vi "JKISM++ Register Status Change.vi"(0 "JKISM Name":string, 5 "Source JKISM Name (* as Default)":string="*", 7 "Status":string, 9 "Response Message (if \"\", same as Source Message)":string, 11 "Error in":errorcluster caption="Error in (no error)", 12 "Priority(T:As Status,F:As Interrupt)":T1) -> (4 "JKISM Name(dup)":string, 15 "Error out":errorcluster)   [LabVIEW 2014, in "JKI State Machine++.lvlib"]
doc: "Register for notification of other JKISM++ Module's status change. If \"Response Message\" is not connected or \"\" is the input, the same state name will be used for acting message.\n\n<b>Inputs:</b>\n - <b>JKISM Name</b>: JKISM Module name.\n - <b>Source JKISM Name (* as Default)</b>: JKISM who generates the status. You can use '*' for all modules generated the same <b>Status</b>\n - <b>Status</b>: The status string\n - <b>Response Message (if \"\", same as Source Message)</b>: After registered, If status change, this message will be received.\n - <b>Priority(T:As Status,F:As Interrupt)</b>: The Response Message will be inserted to the front of state queue if it's False, otherwise it wil be append to the tail.\n - <b>Error in</b>: Error cluster\n\n<b>Outputs:</b>\n - <b>JKISM Name(dup)</b>: Return <b>JKISM Name</b>\n - <b>Error out</b>: Error cluster"
uses:
  JKI State Machine++.lvlib
  JKISM++ Broadcast Message Type.ctl
  _Support/FGV-BroadcastRegistry/Operation-BroadcastRegistry.ctl
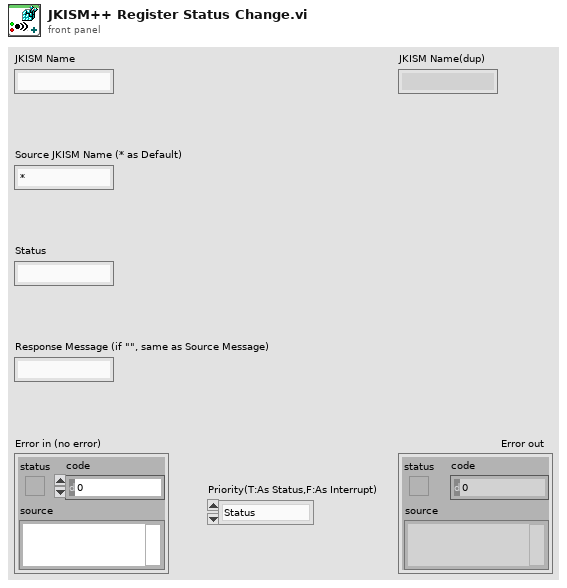
[diagram p1: front panel]
types:
  T1 = typedef "JKI State Machine++.lvlib/JKISM++ Broadcast Message Type.ctl" = enum16{"Status", "Interrupt(High)"}
  T2 = typedef "JKI State Machine++.lvlib/Operation-BroadcastRegistry.ctl" = enum16{"Delete Source Module", "Delete Target Module", "Remove Module", "Register", "Unregister", "Check"}
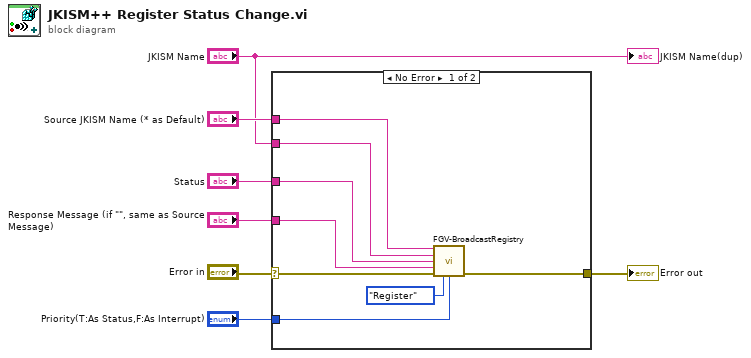
[diagram p0: block diagram]
diagram:
  n1 = case shown="No Error" "Error in" {
    selector: "Error in" -> [w14 w16]
    tunnel: [w13 w16] -> w6
    tunnel: "Response Message (if \"\", same as Source Message)" -> [w12 _]
    tunnel: "Status" -> [w11 _]
    tunnel: "JKISM Name" -> [w10 _]
    tunnel: "Source JKISM Name (* as Default)" -> [w9 _]
    tunnel: "Priority(T:As Status,F:As Interrupt)" -> [w8 _]
    frame No Error {
      n2 = call "FGV-BroadcastRegistry.vi"("Source"=w9, "Target"=w10, "Message"=w11, "Response Message In"=w12, "Error in"=w14, "Operation"=Operation-BroadcastRegistry."Register", "Priority"=w8) -> ("Error out"=w13:errorcluster)  [unwired: 6 in, 2 out]
    }
    frame Error {
    }
  }
  "Error out" <- w6
  "JKISM Name(dup)" <- "JKISM Name"
